vi "Get Gain.vi"(7 "Direction":T1, 8 "error in (no error)":errorcluster, 10 "Index":i32, 11 "VoiceMeeterRemote in":refnum<class "VoiceMeeterRemote.lvclass">) -> (0 "error out":errorcluster, 1 "Value":sgl, 3 "VoiceMeeterRemote out":refnum<class "VoiceMeeterRemote.lvclass">)   [LabVIEW 2020, in "VoiceMeeterRemote.lvlib" / "VoiceMeeterRemote.lvclass"]
doc: "Gets the current gain value for the specified input or output index. The value will be in a range from -60 to +12."
uses:
  VoiceMeeterRemote.lvclass
  Direction.ctl
  VoiceMeeterRemote.lvlib
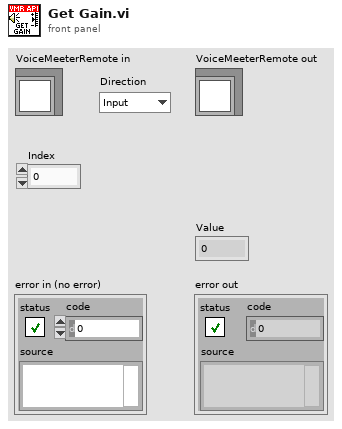
[diagram p1: front panel]
types:
  T1 = typedef "VoiceMeeterRemote.lvlib/Direction.ctl" = enum16{"Input", "Output"}
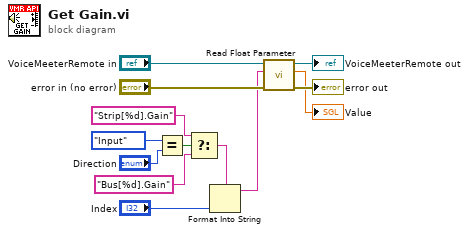
[diagram p0: block diagram]
diagram:
  n1 = Equal?(x=Direction."Input", y="Direction") -> (x = y?=w11:bool)
  n2 = Select(t="Strip[%d].Gain", s=w11, f="Bus[%d].Gain") -> (s? t:f=w8:string)
  n3 = Format Into String(format string=w8, "Index") -> (resulting string=w4:string)  [unwired: 2 in, 1 out]
  n4 = call "Read Float Parameter.vi"("error in (no error)"="error in (no error)", "Parameter Name"=w4, "VoiceMeeterRemote in"="VoiceMeeterRemote in") -> ("error out"=→"error out":errorcluster, "Value"=→"Value":sgl, "VoiceMeeterRemote out"=→"VoiceMeeterRemote out":refnum<class "VoiceMeeterRemote.lvclass">)  [unwired: 6 in]
